vi "Measurement Logic.vi"() -> ()   [LabVIEW 2021, in "Line Transient_Channel Ganging.lvlib"]
uses:
  Line Transient_Channel Ganging.lvlib
  Measurement Results.ctl
  <instrlib>/niDCPower/nidcpower.llb/niDCPower Source Mode.ctl
  <instrlib>/niDCPower/nidcpower.llb/niDCPower Output Function.ctl
  <instrlib>/niDCPower/nidcpower.llb/niDCPower Wait For Event - Event.ctl
  shared subVIs/Triggers and Events/NIDCPower_channel_ganging - Configure Digital Edge Measure Trigger.vi
  shared subVIs/ctl/NIDCPower_channel_ganging - ctl - channel mode.ctl
  <instrlib>/niScope/Controls/niScope trigger slope.ctl
  <instrlib>/niScope/Acquire/Fetch/niScope Fetch WDT.vi
  <instrlib>/niScope/Configure/Trigger/niScope Configure Trigger Digital.vi
  <instrlib>/niScope/Utility/niScope Get Channel Name From String.vi
  shared subVIs/Triggers and Events/NIDCPower_channel_ganging - Configure Digital Edge Source Trigger.vi
  <vilib>/Plug-In SDKs/Measurements/Measure Call Context/Measure Call Context.lvclass
  Measurement Configuration.ctl
panel:
  in  "measurement configuration":T1={"Source master resource name"="", "Load master resource name"="", "Source slave resource names"=[], "Load slave resource names"=[], "Source system configuration"=enum."Parallel", "Source voltage level range"=20.0, "Source limit symmetry"=enum."Asymmetric", "Source current limit range"=25.0, "Source current limit low"=-0.6, "Source current limit high"=25.0, "Source transient response"=1038, "Source sense"=1009, "Source voltage level 1"=6.0, "Source sample rate"=1800000.0, "Source voltage level 2"=14.0, "Source voltage gain bandwidth"=2000.0, "Source voltage compensation frequency"=3530.0, "Source voltage pole-zero ratio"=2.0, "Load system configuration"=enum."Parallel", "Load current level"=1.0, "Load current level range"=80.0, "Load limit symmetry"=enum."Symmetric", "Load voltage limit range"=6.0, "Load voltage limit low"=0.0, "Load voltage limit high"=inf, "Load transient response"=1038, "Load sense"=1009, "DUT setup time"=1.0, "Load current gain bandwidth"=14000.0, "Load current compensation frequency"=180000.0, "Load current pole-zero ratio"=0.3, "Nominal output voltage"=1.0, "Source time delay 1"=6.0, "Source time delay 2"=0.005, "Source pulse duration"=0.005, "Source voltage falling slew rate"=24.0, "Source voltage rising slew rate"=24.0, "Scope resource name"="", "Scope output channel name"="0", "Scope sample rate"=1800000.0, "Scope probe attenuation"=1.0, "Scope vertical range"=10.0, "Scope vertical coupling"=enum."DC", "Scope enable/disable"=TRUE} {"Scope vertical range" format="%.2f"; "Scope probe attenuation" format="%.1f"; "Scope sample rate" step=1000000.0 format="%#.2g"; "Source voltage rising slew rate" format="%#_6p"; "Source time delay 1" format="%#_6p"; "Load sense" items=["Local"=1008, "Remote"=1009]; "Load transient response" items=["Slow"=1041, "Normal"=1038, "Fast"=1039, "Custom"=1042]; "Load voltage limit high" format="%#_6p"; "Load voltage limit low" format="%#_6p"; "Load voltage limit range" format="%#_6p"; "Load current level range" format="%#_6p"; "Source voltage level 1" format="%#_6p"; "Source sense" items=["Local"=1008, "Remote"=1009]; "Source transient response" items=["Slow"=1041, "Normal"=1038, "Fast"=1039, "Custom"=1042]; "Source current limit high" format="%#_6p"; "Source current limit low" format="%#_6p"; "Source current limit range" format="%#_6p"; "Source voltage level range" format="%#_6p"}
  out "measurement results":T2
  out "measure call context out":refnum<class "Measure Call Context.lvclass">
  in  "measure call context in":refnum<class "Measure Call Context.lvclass">
  out "error out":errorcluster
  in  "error in":errorcluster
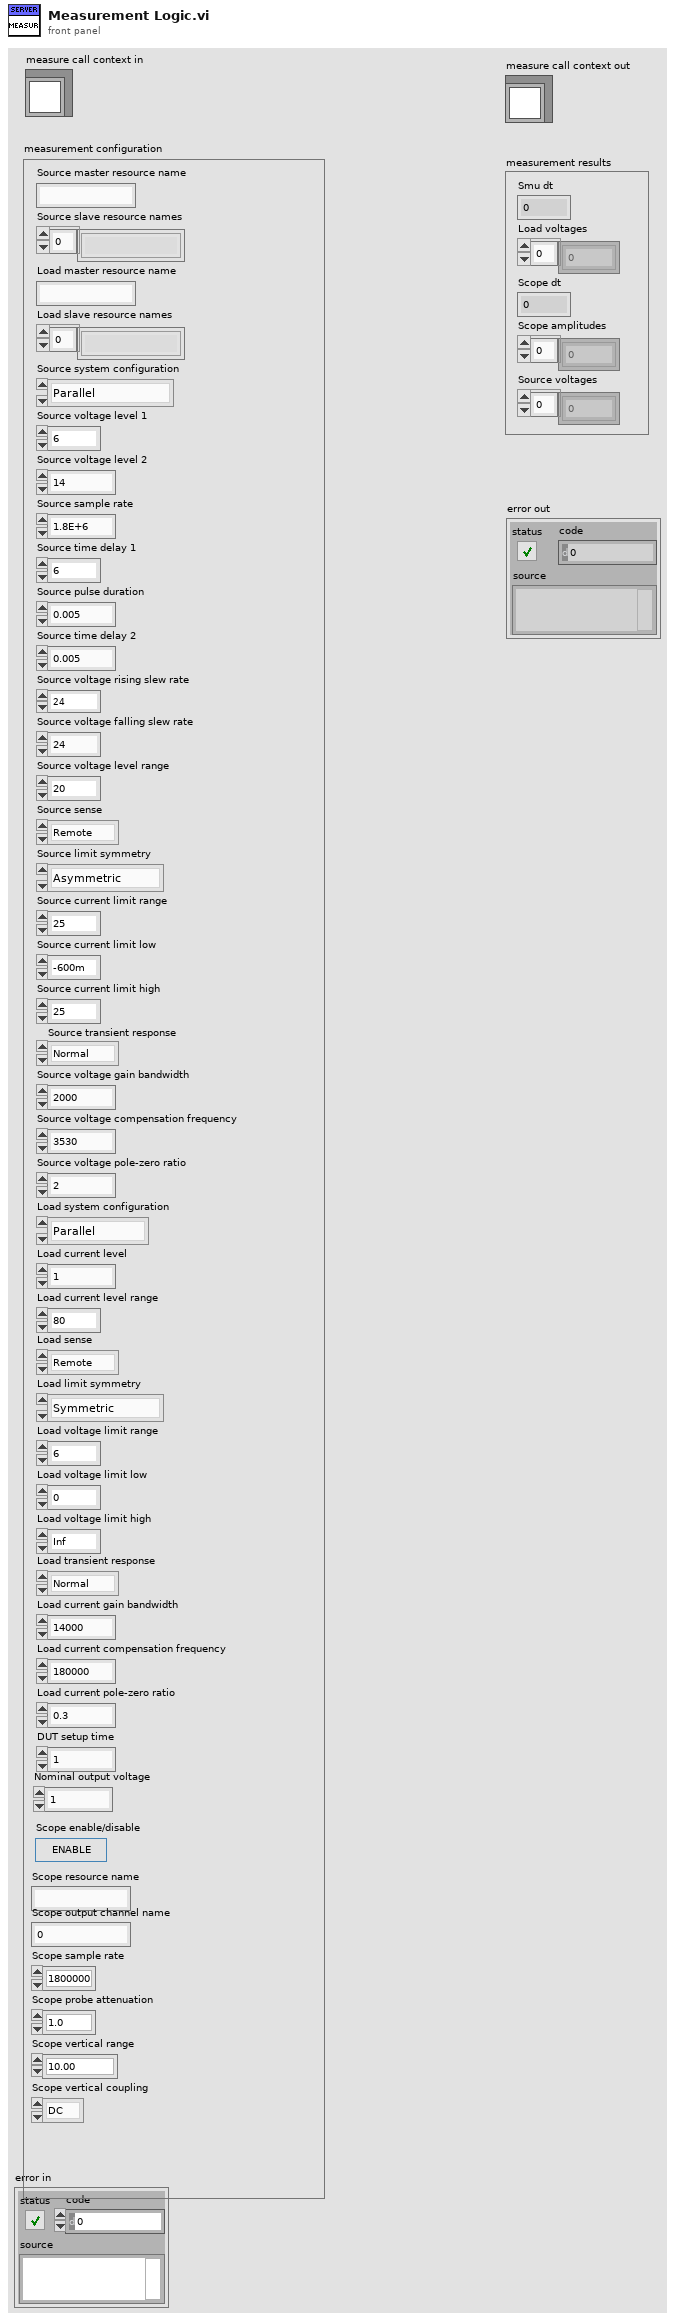
[diagram p1: front panel]
types:
  T1 = typedef "Line Transient_Channel Ganging.lvlib/Measurement Configuration.ctl" = cluster{"Source master resource name":string, "Load master resource name":string, "Source slave resource names":string[], "Load slave resource names":string[], "Source system configuration":enum32{"Series", "Parallel", "Manual"}, "Source voltage level range":dbl, "Source limit symmetry":enum32{"Symmetric", "Asymmetric"}, "Source current limit range":dbl, "Source current limit low":dbl, "Source current limit high":dbl, "Source transient response":i32, "Source sense":i32, "Source voltage level 1":dbl, "Source sample rate":dbl, "Source voltage level 2":dbl, "Source voltage gain bandwidth":dbl, "Source voltage compensation frequency":dbl, "Source voltage pole-zero ratio":dbl, "Load system configuration":enum32{"Series", "Parallel", "Manual"}, "Load current level":dbl, "Load current level range":dbl, "Load limit symmetry":enum32{"Symmetric", "Asymmetric"}, "Load voltage limit range":dbl, "Load voltage limit low":dbl, "Load voltage limit high":dbl, "Load transient response":i32, "Load sense":i32, "DUT setup time":dbl, "Load current gain bandwidth":dbl, "Load current compensation frequency":dbl, "Load current pole-zero ratio":dbl, "Nominal output voltage":dbl, "Source time delay 1":dbl, "Source time delay 2":dbl, "Source pulse duration":dbl, "Source voltage falling slew rate":dbl, "Source voltage rising slew rate":dbl, "Scope resource name":string, "Scope output channel name":string, "Scope sample rate":dbl, "Scope probe attenuation":dbl, "Scope vertical range":dbl, "Scope vertical coupling":enum32{"AC", "DC"}, "Scope enable/disable":bool}
  T2 = typedef "Line Transient_Channel Ganging.lvlib/Measurement Results.ctl" = cluster{"Smu dt":dbl, "Load voltages":dbl[], "Source voltages":dbl[], "Scope amplitudes":dbl[], "Scope dt":dbl}
  T3 = typedef "NIDCPower_channel_ganging - ctl - channel mode.ctl" = enum32{"Master", "Slave", "Slave - Inverted"}
  T4 = typedef "niDCPower Output Function.ctl" = i32
  T5 = typedef "niDCPower Source Mode.ctl" = i32
  T6 = typedef "niDCPower Wait For Event - Event.ctl" = i32
  T7 = typedef "NIDCPower_channel_ganging - ctl - channel def.ctl" = cluster{"resource name":refnum<k15>, "channels":string, "Channel Mode":T3}
  T8 = typedef "NIDCPower_channel_ganging - ctl - ganged session.ctl" = cluster{"Ganged Config":T9, "Session List":refnum<k15>[], "Session Mode":T3[], "Channel":string[]}
  T9 = typedef "NIDCPower_channel_ganging - ctl - ganged config.ctl" = enum32{"Series", "Parallel", "Manual"}
  T10 = typedef "niScope trigger slope.ctl" = i32
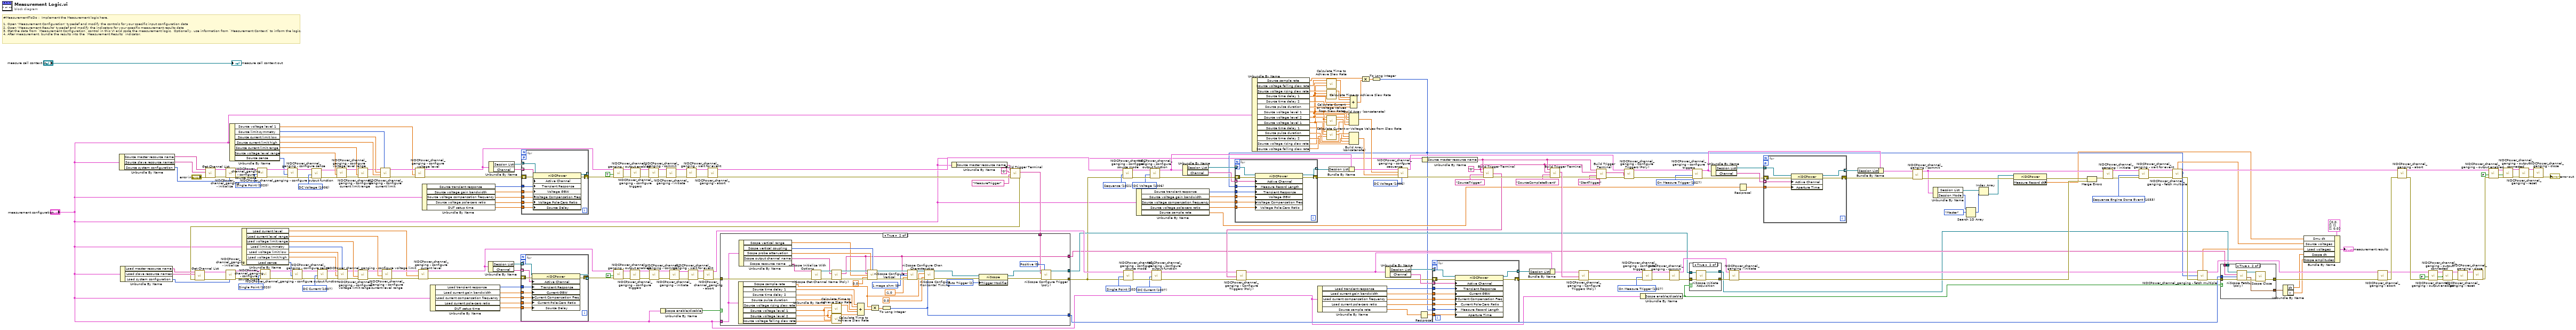
[diagram p0: block diagram]
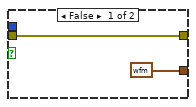
[diagram p2: hidden frame]
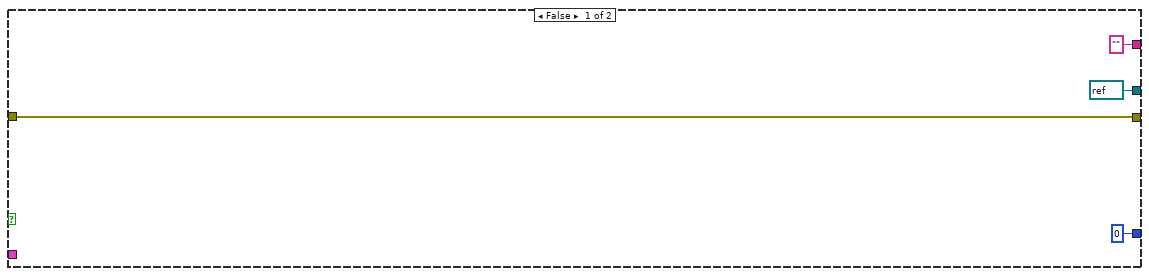
[diagram p4: hidden frame]
diagram:
  w100 = 1027 items=["Automatically after Source Complete"=1025, "On Demand"=1026, "On Measure Trigger"=1027] ("Measure When")
  w113 = T4 1006 items=["DC Voltage"=1006, "DC Current"=1007, "Pulse Voltage"=1049, "Pulse Current"=1050] ("output function")
  w96 = "0" ("Channel Name")
  w141 = 1027 items=["Automatically after Source Complete"=1025, "On Demand"=1026, "On Measure Trigger"=1027] ("Measure When")
  w138 = T4 1006 items=["DC Voltage"=1006, "DC Current"=1007, "Pulse Voltage"=1049, "Pulse Current"=1050] ("output function")
  w142 = T5 1021 items=["Single Point"=1020, "Sequence"=1021] ("source mode")
  w19 = T5 1020 items=["Single Point"=1020, "Sequence"=1021] ("source mode")
  w118 = T4 1007 items=["DC Voltage"=1006, "DC Current"=1007, "Pulse Voltage"=1049, "Pulse Current"=1050] ("output function")
  w147 = T6 1033 items=["Source Complete Event"=1030, "Measure Complete Event"=1031, "Sequence Iteration Complete Event"=1032, "Sequence Engine Done Event"=1033, "Pulse Complete Event"=1051, "Ready For Pulse Trigger Event"=1052] ("event")
  w151 = FALSE ("output enabled")
  w150 = FALSE ("output enabled")
  w223 = T4 1007 items=["DC Voltage"=1006, "DC Current"=1007, "Pulse Voltage"=1049, "Pulse Current"=1050] ("output function")
  w236 = T4 1006 items=["DC Voltage"=1006, "DC Current"=1007, "Pulse Voltage"=1049, "Pulse Current"=1050] ("output function")
  w255 = T5 1020 items=["Single Point"=1020, "Sequence"=1021] ("source mode")
  w256 = T5 1020 items=["Single Point"=1020, "Sequence"=1021] ("source mode")
  # "#MeasurementToDo :  Implement the Measurement logic here.\n\n1. Open 'Measurement Configuration' typedef and modify the controls for your specific input configuration data\n2. Open 'Measurement Results' typedef and modify the indicators for your specific measurement results data\n3. Get the data from `Measurement Configuration` control in this VI and code the measurement logic.  Optionally, use information from `Measurement Context` to inform the logic.\n4. After measurement, bundle the results into the `Measurement Results` indicator."
  n1 = Unbundle By Name("measurement configuration") -> ("Source master resource name"=w178:string, "Source slave resource names"=w177:string[], "Source system configuration"=w238:enum32{"Series", "Parallel", "Manual"})
  n2 = Unbundle By Name("measurement configuration") -> ("Load master resource name"=w174:string, "Load slave resource names"=w173:string[], "Load system configuration"=w237:enum32{"Series", "Parallel", "Manual"})
  n3 = call "Get Channel List.vi"("error in (no error)"="error in", "Slave resource names"=w177, "Master resouce name"=w178) -> ("error out"=w179:errorcluster, "Channel List"=w180:T7[])  [unwired: 7 in]
  n4 = call "NIDCPower_channel_ganging - initialize.vi"("Ganged Config"=w238, "error in (no error)"=w179, "Channel List"=w180) -> ("error out"=w257:errorcluster, "Ganged Session Out"=w258:T8)  [unwired: 7 in]
  n5 = Unbundle By Name("measurement configuration") -> ("Source voltage level 1"=w94:dbl, "Source limit symmetry"=w244:enum32{"Symmetric", "Asymmetric"}, "Source current limit low"=w245:dbl, "Source current limit high"=w246:dbl, "Source current limit range"=w247:dbl, "Source voltage level range"=w248:dbl, "Source sense"=w181:i32)
  n6 = Unbundle By Name("measurement configuration") -> ("Load current level"=w183:dbl, "Load current level range"=w239:dbl, "Load voltage limit range"=w240:dbl, "Load limit symmetry"=w243:enum32{"Symmetric", "Asymmetric"}, "Load voltage limit low"=w242:dbl, "Load voltage limit high"=w241:dbl, "Load sense"=w182:i32)
  n7 = call "NIDCPower_channel_ganging - configure source mode.vi"("error in (no error)"=w257, "source mode"=w256, "Ganged Session In"=w258) -> ("error out"=w221:errorcluster, "Ganged Session Out"=w222:T8)  [unwired: 7 in]
  n8 = call "NIDCPower_channel_ganging - configure sense.vi"("error in (no error)"=w221, "sense"=w181, "Ganged Session In"=w222) -> ("error out"=w219:errorcluster, "Ganged Session Out"=w220:T8)  [unwired: 7 in]
  n9 = call "NIDCPower_channel_ganging - configure output function.vi"("error in (no error)"=w219, "output function"=w236, "Ganged Session In"=w220) -> ("error out"=w217:errorcluster, "Ganged Session Out"=w218:T8)  [unwired: 7 in]
  n10 = call "NIDCPower_channel_ganging - configure voltage level range.vi"("error in (no error)"=w217, "voltage level range"=w248, "Ganged Session In"=w218) -> ("error out"=w232:errorcluster, "Ganged Session Out"=w235:T8)  [unwired: 7 in]
  n11 = call "NIDCPower_channel_ganging - configure current limit range.vi"("error in (no error)"=w232, "current limit range"=w247, "Ganged Session In"=w235) -> ("error out"=w231:errorcluster, "Ganged Session Out"=w234:T8)  [unwired: 7 in]
  n12 = call "NIDCPower_channel_ganging - configure current limit.vi"("Limit Symmetry"=w244, "error in (no error)"=w231, "Current limit/hi"=w246, "Current limit lo"=w245, "Ganged Session In"=w234) -> ("error out"=w230:errorcluster, "Ganged Session Out"=w233:T8)  [unwired: 5 in]
  n13 = call "NIDCPower_channel_ganging - configure voltage level.vi"("error in (no error)"=w230, "voltage level"=w94, "Ganged Session In"=w233) -> ("error out"=w192:errorcluster, "Ganged Session Out"=w186:T8)  [unwired: 7 in]
  n14 = Unbundle By Name("measurement configuration") -> ("Source transient response"=w172:i32, "Source voltage gain bandwidth"=w168:dbl, "Source voltage compensation frequency"=w167:dbl, "Source voltage pole-zero ratio"=w166:dbl, "DUT setup time"=w169:dbl)
  n15 = Unbundle By Name("measurement configuration") -> ("Load transient response"=w171:i32, "Load current gain bandwidth"=w165:dbl, "Load current compensation frequency"=w164:dbl, "Load current pole-zero ratio"=w163:dbl, "DUT setup time"=w170:dbl)
  n16 = Unbundle By Name(w186) -> ("Session List"=w190:refnum<k15>[], "Channel"=w189:string[])
  n17 = for {
    tunnel: [w269] -> _ mode=indexing
    shift-right: [w267] -> w191
    shift-left: w192 -> [w268]
    workers-P: _ -> [_]
    tunnel: w190 -> [w266] mode=indexing
    tunnel: w189 -> [w265] mode=indexing
    tunnel: w172 -> [w264]
    tunnel: w169 -> [w263]
    tunnel: w168 -> [w262]
    tunnel: w167 -> [w261]
    tunnel: w166 -> [w260]
    n18 = property class="niDCPower"(reference=w266, error in=w268, "Active Channel"=w265, "Transient Response"=w264, "Voltage GBW"=w262, "Voltage Compensation Freq"=w261, "Voltage Pole-Zero Ratio"=w260, "Source Delay"=w263) -> (reference out=w269:refnum<k15>, error out=w267:errorcluster)
  }
  n19 = call "NIDCPower_channel_ganging - output enabled.vi"("error in (no error)"=w191, "output enabled"=TRUE, "Ganged Session In"=w186) -> ("error out"=w195:errorcluster, "Ganged Session Out"=w196:T8)  [unwired: 7 in]
  n20 = call "NIDCPower_channel_ganging - configure triggers.vi"("error in (no error)"=w195, "Ganged Session In"=w196) -> ("error out"=w193:errorcluster, "Ganged Session Out"=w194:T8)  [unwired: 8 in]
  n21 = call "NIDCPower_channel_ganging - commit.vi"("error in (no error)"=w193, "Ganged Session In"=w194) -> ("error out"=w202:errorcluster, "Ganged Session Out"=w201:T8)  [unwired: 8 in]
  n22 = Unbundle By Name("measurement configuration") -> ("Scope enable/disable"=w13:bool)
  n23 = call "NIDCPower_channel_ganging - initiate.vi"("error in (no error)"=w202, "Ganged Session In"=w201) -> ("error out"=w204:errorcluster, "Ganged Session Out"=w203:T8)  [unwired: 8 in]
  n24 = call "NIDCPower_channel_ganging - wait for event.vi"("error in (no error)"=w204, "Ganged Session in"=w203) -> ("error out"=w206:errorcluster, "Ganged Session Out"=w205:T8)  [unwired: 8 in]
  n25 = call "NIDCPower_channel_ganging - abort.vi"("error in (no error)"=w206, "Ganged Session In"=w205) -> ("error out"=w33:errorcluster, "Ganged Session Out"=w31:T8)  [unwired: 8 in]
  n26 = Unbundle By Name("measurement configuration") -> ("Source master resource name"=w30:string)
  n27 = call "Build Trigger Terminal.vi"("error in (no error)"=w33, "Trigger/Event Name"="MeasureTrigger", "Channel Name"="0", "Resource Name"=w30) -> ("error out"=w34:errorcluster, "Terminal Name"=w18:string)  [unwired: 6 in]
  n28 = call "Get Channel List.vi"("error in (no error)"=w34, "Slave resource names"=w173, "Master resouce name"=w174) -> ("error out"=w176:errorcluster, "Channel List"=w175:T7[])  [unwired: 7 in]
  n29 = call "NIDCPower_channel_ganging - initialize.vi"("Ganged Config"=w237, "error in (no error)"=w176, "Channel List"=w175) -> ("error out"=w254:errorcluster, "Ganged Session Out"=w253:T8)  [unwired: 7 in]
  n30 = call "NIDCPower_channel_ganging - configure source mode.vi"("error in (no error)"=w254, "source mode"=w255, "Ganged Session In"=w253) -> ("error out"=w215:errorcluster, "Ganged Session Out"=w216:T8)  [unwired: 7 in]
  n31 = call "NIDCPower_channel_ganging - configure sense.vi"("error in (no error)"=w215, "sense"=w182, "Ganged Session In"=w216) -> ("error out"=w213:errorcluster, "Ganged Session Out"=w214:T8)  [unwired: 7 in]
  n32 = call "NIDCPower_channel_ganging - configure output function.vi"("error in (no error)"=w213, "output function"=w223, "Ganged Session In"=w214) -> ("error out"=w251:errorcluster, "Ganged Session Out"=w252:T8)  [unwired: 7 in]
  n33 = call "NIDCPower_channel_ganging - configure voltage limit.vi"("Limit Symmetry"=w243, "error in (no error)"=w251, "voltage limit/hi"=w241, "voltage limit lo"=w242, "Ganged Session In"=w252) -> ("error out"=w228:errorcluster, "Ganged Session Out"=w229:T8)  [unwired: 5 in]
  n34 = call "NIDCPower_channel_ganging - configure voltage limit range.vi"("error in (no error)"=w228, "voltage level range"=w240, "Ganged Session In"=w229) -> ("error out"=w226:errorcluster, "Ganged Session Out"=w227:T8)  [unwired: 7 in]
  n35 = call "NIDCPower_channel_ganging - configure current level range.vi"("error in (no error)"=w226, "current level range"=w239, "Ganged Session In"=w227) -> ("error out"=w224:errorcluster, "Ganged Session Out"=w225:T8)  [unwired: 7 in]
  n36 = call "NIDCPower_channel_ganging - configure current level.vi"("error in (no error)"=w224, "current level"=w183, "Ganged Session In"=w225) -> ("error out"=w188:errorcluster, "Ganged Session Out"=w60:T8)  [unwired: 7 in]
  n37 = Unbundle By Name(w60) -> ("Session List"=w185:refnum<k15>[], "Channel"=w184:string[])
  n38 = for {
    tunnel: [w279] -> _ mode=indexing
    shift-right: [w277] -> w187
    shift-left: w188 -> [w278]
    workers-P: _ -> [_]
    tunnel: w185 -> [w276] mode=indexing
    tunnel: w184 -> [w275] mode=indexing
    tunnel: w171 -> [w274]
    tunnel: w170 -> [w273]
    tunnel: w165 -> [w272]
    tunnel: w164 -> [w271]
    tunnel: w163 -> [w270]
    n39 = property class="niDCPower"(reference=w276, error in=w278, "Active Channel"=w275, "Transient Response"=w274, "Current GBW"=w272, "Current Compensation Freq"=w271, "Current Pole-Zero Ratio"=w270, "Source Delay"=w273) -> (reference out=w279:refnum<k15>, error out=w277:errorcluster)
  }
  n40 = call "NIDCPower_channel_ganging - output enabled.vi"("error in (no error)"=w187, "output enabled"=TRUE, "Ganged Session In"=w60) -> ("error out"=w199:errorcluster, "Ganged Session Out"=w200:T8)  [unwired: 7 in]
  n41 = call "NIDCPower_channel_ganging - configure triggers.vi"("error in (no error)"=w199, "Ganged Session In"=w200) -> ("error out"=w197:errorcluster, "Ganged Session Out"=w198:T8)  [unwired: 8 in]
  n42 = call "NIDCPower_channel_ganging - commit.vi"("error in (no error)"=w197, "Ganged Session In"=w198) -> ("error out"=w211:errorcluster, "Ganged Session Out"=w212:T8)  [unwired: 8 in]
  n43 = call "NIDCPower_channel_ganging - initiate.vi"("error in (no error)"=w211, "Ganged Session In"=w212) -> ("error out"=w209:errorcluster, "Ganged Session Out"=w210:T8)  [unwired: 8 in]
  n44 = call "NIDCPower_channel_ganging - wait for event.vi"("error in (no error)"=w209, "Ganged Session in"=w210) -> ("error out"=w207:errorcluster, "Ganged Session Out"=w208:T8)  [unwired: 8 in]
  n45 = call "NIDCPower_channel_ganging - abort.vi"("error in (no error)"=w207, "Ganged Session In"=w208) -> ("error out"=w20:errorcluster, "Ganged Session Out"=w105:T8)  [unwired: 8 in]
  n46 = case shown="True" w13 {
    tunnel: w20 -> [w283 w293]
    tunnel: "measurement configuration" -> [_ w292]
    tunnel: [w283 w291] -> w2
    tunnel: w18 -> [_ w290]
    tunnel: ["" ("channel name") w288] -> w16
    tunnel: [refnum<k15> refnum ("instrument handle out") w287] -> w17
    tunnel: [0 w286] -> w14
    frame False {
    }
    frame True {
      w314 = 2 items=["None"=1, "Auto Trigger"=2] ("Trigger Modifier")
      w307 = u32 0 items=["1 mega ohm"=0, "50 ohms"=2] ("Input Impedance")
      w311 = T10 0 items=["Positive", "Negative"] ("trigger slope")
      n47 = Unbundle By Name(w292) -> ("Scope sample rate"=w284:dbl, "Source time delay 1"=w305:dbl, "Source time delay 2"=w304:dbl, "Source pulse duration"=w303:dbl, "Source voltage rising slew rate"=w301:dbl, "Source voltage level 1"=w296:dbl, "Source voltage level 2"=w297:dbl, "Source voltage falling slew rate"=w299:dbl)
      n48 = Unbundle By Name(w292) -> ("Scope vertical range"=w285:dbl, "Scope vertical coupling"=w309:enum32{"AC", "DC"}, "Scope probe attenuation"=w310:dbl, "Scope output channel name"=w308:string, "Scope resource name"=w289:string)
      n49 = call <instrlib>:"niScope Initialize With Options.vi"("resource name"=w289, "error in"=w293) -> ("instrument handle"=w325:refnum<k15>, "error out"=w324:errorcluster)  [unwired: 12 in]
      n50 = call-poly <instrlib>:"niScope Get Channel Name (Poly).vi"("instrument handle"=w325, "index"=w308, "error in"=w324) -> ("instrument handle out"=w313:refnum<k15>, "channel name"=w288:string, "error out"=w312:errorcluster)  [unwired: 10 in]
      n51 = call "Calculate Time to Achieve Slew Rate.vi"("Current/voltage set point 2"=w297, "Current/voltage set point 1"=w296, "Current/voltage slew rate"=w301) -> ("Calculated time"=w300:dbl)  [unwired: 8 in]
      n52 = call "Calculate Time to Achieve Slew Rate.vi"("Current/voltage set point 2"=w296, "Current/voltage set point 1"=w297, "Current/voltage slew rate"=w299) -> ("Calculated time"=w298:dbl)  [unwired: 8 in]
      n53 = Compound Arithmetic op=ADD(w305, w304, w303, w300, w298) -> (w294:dbl)
      n54 = call <instrlib>:"niScope Configure Vertical.vi"("instrument handle"=w313, "probe attenuation"=w310, "vertical coupling"=w309, "channels"=w288, "vertical range"=w285, "vertical offset"=0.0, "error in"=w312) -> ("instrument handle out"=w323:refnum<k15>, "error out"=w322:errorcluster)  [unwired: 7 in]
      n55 = Compound Arithmetic op=MULTIPLY(w284, w294) -> (w295:dbl)
      n56 = To Long Integer(number=w295) -> (32bit integer=w286:i32)
      n57 = call <instrlib>:"niScope Configure Chan Characteristics.vi"("instrument handle"=w323, "channels"=w288, "input impedance"=w307, "maximum input frequency"=-1.0 ("Maximum Input Frequency"), "error in"=w322) -> ("instrument handle out"=w320:refnum<k15>, "error out"=w321:errorcluster)  [unwired: 9 in]
      n58 = call <instrlib>:"niScope Configure Horizontal Timing.vi"("instrument handle"=w320, "min sample rate"=w284, "reference position"=0.0 ("Reference Position"), "error in"=w321, "min record length"=w286) -> ("instrument handle out"=w317:refnum<k15>, "error out"=w316:errorcluster)  [unwired: 9 in]
      n59 = property on="Property Node" class="niScope"(reference=w317, error in=w316, "Trigger Modifier"=w314) -> (reference out=w302:refnum<k15>, error out=w315:errorcluster)
      n60 = call-poly <instrlib>:"niScope Configure Trigger (poly).vi"("instrument handle"=w302, "trigger slope"=w311, "trigger source"=w290, "error in"=w315) -> ("instrument handle out"=w287:refnum<k15>, "error out"=w291:errorcluster)  [unwired: 10 in]
    }
  }
  n61 = call "NIDCPower_channel_ganging - configure source mode.vi"("error in (no error)"=w2, "source mode"=w142, "Ganged Session In"=w31) -> ("error out"=w143:errorcluster, "Ganged Session Out"=w144:T8)  [unwired: 7 in]
  n62 = call "NIDCPower_channel_ganging - configure source mode.vi"("error in (no error)"=w2, "source mode"=w19, "Ganged Session In"=w105) -> ("error out"=w146:errorcluster, "Ganged Session Out"=w145:T8)  [unwired: 7 in]
  n63 = Unbundle By Name("measurement configuration") -> ("Source transient response"=w114:i32, "Source voltage gain bandwidth"=w111:dbl, "Source voltage compensation frequency"=w110:dbl, "Source voltage pole-zero ratio"=w109:dbl, "Source sample rate"=w24:dbl)
  n64 = call "NIDCPower_channel_ganging - configure output function.vi"("error in (no error)"=w143, "output function"=w138, "Ganged Session In"=w144) -> ("error out"=w139:errorcluster, "Ganged Session Out"=w140:T8)  [unwired: 7 in]
  n65 = call "NIDCPower_channel_ganging - configure output function.vi"("error in (no error)"=w146, "output function"=w118, "Ganged Session In"=w145) -> ("error out"=w55:errorcluster, "Ganged Session Out"=w53:T8)  [unwired: 7 in]
  n66 = Unbundle By Name(w140) -> ("Session List"=w162:refnum<k15>[], "Channel"=w128:string[])
  n67 = Unbundle By Name("measurement configuration") -> ("Source sample rate"=w86:dbl, "Source voltage falling slew rate"=w84:dbl, "Source voltage rising slew rate"=w82:dbl, "Source time delay 1"=w92:dbl, "Source time delay 2"=w85:dbl, "Source pulse duration"=w90:dbl, "Source voltage level 1"=w80:dbl, "Source voltage level 2"=w76:dbl, "Source voltage level 1"=w75:dbl, "Source time delay 1"=w89:dbl, "Source pulse duration"=w88:dbl, "Source time delay 2"=w87:dbl, "Source voltage rising slew rate"=w79:dbl, "Source voltage falling slew rate"=w74:dbl)
  n68 = Unbundle By Name("measurement configuration") -> ("Load transient response"=w112:i32, "Load current gain bandwidth"=w108:dbl, "Load current compensation frequency"=w107:dbl, "Load current pole-zero ratio"=w106:dbl, "Source sample rate"=w59:dbl)
  n69 = call "Calculate Time to Achieve Slew Rate.vi"("Current/voltage set point 2"=w80, "Current/voltage set point 1"=w76, "Current/voltage slew rate"=w84) -> ("Calculated time"=w83:dbl)  [unwired: 8 in]
  n70 = call "Calculate Time to Achieve Slew Rate.vi"("Current/voltage set point 2"=w76, "Current/voltage set point 1"=w80, "Current/voltage slew rate"=w82) -> ("Calculated time"=w81:dbl)  [unwired: 8 in]
  n71 = call "Calculate Current or Voltage Values from Slew Rate.vi"("Current/voltage slew rate"=w79, "Current/voltage end point"=w76, "Current/voltage start point"=w80) -> ("Source delays"=w77:dbl[], "Current/voltage values"=w78:dbl[])  [unwired: 7 in]
  n72 = call "Calculate Current or Voltage Values from Slew Rate.vi"("Current/voltage slew rate"=w74, "Current/voltage end point"=w75, "Current/voltage start point"=w76) -> ("Source delays"=w72:dbl[], "Current/voltage values"=w73:dbl[])  [unwired: 7 in]
  n73 = Build Array (concatenate)(w80, w78, w76, w73, w75) -> (w71:dbl[])
  n74 = Build Array (concatenate)(w89, w77, w88, w72, w87) -> (w70:dbl[])
  n75 = Compound Arithmetic op=ADD(w83, w81, w92, w85, w90) -> (w91:dbl)
  n76 = Compound Arithmetic op=MULTIPLY(w86, w91) -> (w93:dbl)
  n77 = To Long Integer(number=w93) -> (32bit integer=w3:i32)
  n78 = for {
    tunnel: [w335] -> w161 mode=indexing
    shift-right: [w333] -> w116
    shift-left: w139 -> [w334]
    workers-P: _ -> [_]
    tunnel: w162 -> [w332] mode=indexing
    tunnel: w128 -> [w327] mode=indexing
    tunnel: w114 -> [w331]
    tunnel: w111 -> [w330]
    tunnel: w110 -> [w329]
    tunnel: w109 -> [w328]
    tunnel: w3 -> [w326]
    n79 = property class="niDCPower"(reference=w332, error in=w334, "Active Channel"=w327, "Measure Record Length"=w326, "Transient Response"=w331, "Voltage GBW"=w330, "Voltage Compensation Freq"=w329, "Voltage Pole-Zero Ratio"=w328) -> (reference out=w335:refnum<k15>, error out=w333:errorcluster)
  }
  n80 = Bundle By Name(cluster=w140, "Session List"=w161) -> (w117:T8)
  n81 = call "NIDCPower_channel_ganging - confgure sequence.vi"("output function"=w113, "error in (no error)"=w116, "Source Delays"=w70, "Values"=w71, "Ganged Session In"=w117) -> ("error out"=w115:errorcluster, "Ganged Session Out"=w102:T8)  [unwired: 5 in]
  n82 = Reciprocal(x=w59) -> (1/x=w58:dbl)
  n83 = Unbundle By Name("measurement configuration") -> ("Source master resource name"=w97:string)
  n84 = call "Build Trigger Terminal.vi"("error in (no error)"=w115, "Trigger/Event Name"="SourceTrigger", "Channel Name"=w96, "Resource Name"=w97) -> ("error out"=w124:errorcluster, "Terminal Name"=w51:string)  [unwired: 6 in]
  n85 = call-poly "NIDCPower_channel_ganging - Configure Triggers (Poly).vi"("error in (no error)"=w55, "output terminal"=w51, "Ganged Session in"=w53) -> ("error out"=w54:errorcluster, "Ganged Session out"=w52:T8)  [unwired: 7 in]
  n86 = Unbundle By Name(w52) -> ("Session List"=w127:refnum<k15>[], "Channel"=w126:string[])
  n87 = for {
    tunnel: [w346] -> w125 mode=indexing
    shift-right: [w344] -> w57
    shift-left: w54 -> [w345]
    workers-P: _ -> [_]
    tunnel: w127 -> [w343] mode=indexing
    tunnel: w126 -> [w342] mode=indexing
    tunnel: w112 -> [w341]
    tunnel: w108 -> [w340]
    tunnel: w107 -> [w339]
    tunnel: w106 -> [w338]
    tunnel: w3 -> [w337]
    tunnel: w58 -> [w336]
    n88 = property class="niDCPower"(reference=w343, error in=w345, "Active Channel"=w342, "Transient Response"=w341, "Current GBW"=w340, "Current Compensation Freq"=w339, "Current Pole-Zero Ratio"=w338, "Measure Record Length"=w337, "Aperture Time"=w336) -> (reference out=w346:refnum<k15>, error out=w344:errorcluster)
  }
  n89 = Bundle By Name(cluster=w52, "Session List"=w125) -> (w56:T8)
  n90 = call "Build Trigger Terminal.vi"("error in (no error)"=w124, "Trigger/Event Name"="SourceCompleteEvent", "Channel Name"=w96, "Resource Name"=w97) -> ("error out"=w99:errorcluster, "Terminal Name"=w119:string)  [unwired: 6 in]
  n91 = call-poly "NIDCPower_channel_ganging - Configure Triggers (Poly).vi"("error in (no error)"=w57, "output terminal"=w119, "Ganged Session in"=w56) -> ("error out"=w120:errorcluster, "Ganged Session out"=w121:T8)  [unwired: 7 in]
  n92 = call "Build Trigger Terminal.vi"("error in (no error)"=w99, "Trigger/Event Name"="StartTrigger" ("Source master resource name"), "Channel Name"=w96, "Resource Name"=w97) -> ("error out"=w104:errorcluster, "Terminal Name"=w95:string)  [unwired: 6 in]
  n93 = call-poly "NIDCPower_channel_ganging - Configure Triggers (Poly).vi"("error in (no error)"=w104, "output terminal"=w95, "Ganged Session in"=w102) -> ("error out"=w103:errorcluster, "Ganged Session out"=w101:T8)  [unwired: 7 in]
  n94 = Unbundle By Name("measurement configuration") -> ("Scope enable/disable"=w12:bool)
  n95 = call "NIDCPower_channel_ganging - configure triggers.vi"("error in (no error)"=w120, "Measure When"=w141, "Ganged Session In"=w121) -> ("error out"=w37:errorcluster, "Ganged Session Out"=w36:T8)  [unwired: 7 in]
  n96 = call "NIDCPower_channel_ganging - commit.vi"("error in (no error)"=w37, "Ganged Session In"=w36) -> ("error out"=w28:errorcluster, "Ganged Session Out"=w35:T8)  [unwired: 8 in]
  n97 = case shown="True" w12 {
    tunnel: w28 -> [w347 w350]
    tunnel: [w347 w351] -> w27
    tunnel: w17 -> [_ w349]
    tunnel: [_ w348] -> w15
    frame False {
    }
    frame True {
      n98 = call <instrlib>:"niScope Initiate Acquisition.vi"("instrument handle"=w349, "error in"=w350) -> ("instrument handle out"=w348:refnum<k15>, "error out"=w351:errorcluster)  [unwired: 12 in]
    }
  }
  n99 = call "NIDCPower_channel_ganging - configure triggers.vi"("error in (no error)"=w103, "Measure When"=w100, "Ganged Session In"=w101) -> ("error out"=w65:errorcluster, "Ganged Session Out"=w66:T8)  [unwired: 7 in]
  n100 = Unbundle By Name(w66) -> ("Session List"=w69:refnum<k15>[], "Channel"=w67:string[])
  n101 = call "NIDCPower_channel_ganging - initiate.vi"("error in (no error)"=w27, "Ganged Session In"=w35) -> ("error out"=w148:errorcluster, "Ganged Session Out"=w50:T8)  [unwired: 8 in]
  n102 = Reciprocal(x=w24) -> (1/x=w23:dbl)
  n103 = for {
    tunnel: [w352] -> w68 mode=indexing
    shift-right: [w356] -> w41
    shift-left: w65 -> [w357]
    workers-P: _ -> [_]
    tunnel: w69 -> [w355] mode=indexing
    tunnel: w67 -> [w354] mode=indexing
    tunnel: w23 -> [w353]
    n104 = property class="niDCPower"(reference=w355, error in=w357, "Active Channel"=w354, "Aperture Time"=w353) -> (reference out=w352:refnum<k15>, error out=w356:errorcluster)
  }
  n105 = Bundle By Name(cluster=w66, "Session List"=w68) -> (w40:T8)
  n106 = call "NIDCPower_channel_ganging - commit.vi"("error in (no error)"=w41, "Ganged Session In"=w40) -> ("error out"=w47:errorcluster, "Ganged Session Out"=w39:T8)  [unwired: 8 in]
  n107 = Unbundle By Name(w39) -> ("Session List"=w45:refnum<k15>[], "Session Mode"=w44:T3[])
  n108 = Search 1D Array(1D array=w44, element=NIDCPower_channel_ganging_-_ctl_-_channel_mode."Master") -> (index of element=w42:i32)  [unwired: 1 in]
  n109 = Index Array(array=w45, index=w42) -> (element=w46:refnum<k15>)
  n110 = property class="niDCPower"(reference=w46, error in=w47) -> (error out=w38:errorcluster, "Measure Record dt"=w9:dbl)  [unwired: 1 out]
  n111 = Merge Errors(w38, w148) -> (w149:errorcluster)
  n112 = call "NIDCPower_channel_ganging - initiate.vi"("error in (no error)"=w149, "Ganged Session In"=w39) -> ("error out"=w137:errorcluster, "Ganged Session Out"=w49:T8)  [unwired: 8 in]
  n113 = call "NIDCPower_channel_ganging - wait for event.vi"("error in (no error)"=w137, "event"=w147, "Ganged Session in"=w49) -> ("error out"=w63:errorcluster, "Ganged Session Out"=w48:T8)  [unwired: 7 in]
  n114 = call "NIDCPower_channel_ganging - fetch multiple.vi"("Ganged Session In"=w48, "Count"=w3, "error in (no error)"=w63) -> ("Ganged Voltage Measurement"=w4:dbl[], "Ganged Session Out"=w64:T8, "error out"=w62:errorcluster)  [unwired: 5 in, 5 out]
  n115 = call "NIDCPower_channel_ganging - fetch multiple.vi"("Ganged Session In"=w50, "Count"=w3, "error in (no error)"=w62) -> ("Ganged Voltage Measurement"=w8:dbl[], "Ganged Session Out"=w61:T8, "error out"=w26:errorcluster)  [unwired: 5 in, 5 out]
  n116 = case shown="True" w12 {
    tunnel: w26 -> [w359 w367]
    tunnel: [w359 w366] -> w25
    tunnel: w16 -> [_ w363]
    tunnel: w15 -> [_ w362]
    tunnel: w14 -> [_ w361]
    tunnel: [waveform(dbl) {"t0"=timestamp(0 s since 1904-01-01), "dt"=1.0, "Y"=[]} ("wfm") w360] -> w7
    frame False {
    }
    frame True {
      n117 = call-poly <instrlib>:"niScope Fetch (poly).vi"("error in"=w367, "numSamples"=w361, "channels"=w363, "instrument handle"=w362) -> ("error out"=w365:errorcluster, "wfm"=w360:waveform(dbl), "instrument handle out"=w364:refnum<k15>)  [unwired: 4 in, 1 out]
      n118 = call <instrlib>:"niScope Close.vi"("instrument handle"=w364, "error in"=w365) -> ("error out"=w366:errorcluster)  [unwired: 13 in]
    }
  }
  n119 = Unbundle By Name(w7) -> ("dt"=w6:dbl, "Y"=w5:dbl[])
  n120 = Bundle By Name(cluster=T2 {"Smu dt"=0.0, "Load voltages"=[], "Source voltages"=[], "Scope amplitudes"=[], "Scope dt"=0.0} ("Measurement Results"), "Smu dt"=w9, "Source voltages"=w4, "Load voltages"=w8, "Scope dt"=w6, "Scope amplitudes"=w5) -> (→"measurement results":T2)
  n121 = call "NIDCPower_channel_ganging - abort.vi"("error in (no error)"=w25, "Ganged Session In"=w61) -> ("error out"=w160:errorcluster, "Ganged Session Out"=w156:T8)  [unwired: 8 in]
  n122 = call "NIDCPower_channel_ganging - abort.vi"("error in (no error)"=w160, "Ganged Session In"=w64) -> ("error out"=w159:errorcluster, "Ganged Session Out"=w152:T8)  [unwired: 8 in]
  n123 = call "NIDCPower_channel_ganging - output enabled.vi"("error in (no error)"=w159, "output enabled"=w151, "Ganged Session In"=w156) -> ("error out"=w157:errorcluster, "Ganged Session Out"=w158:T8)  [unwired: 7 in]
  n124 = call "NIDCPower_channel_ganging - output connected.vi"("error in (no error)"=w157, "output enabled"=w151, "Ganged Session In"=w158) -> ("error out"=w136:errorcluster, "Ganged Session Out"=w135:T8)  [unwired: 7 in]
  n125 = call "NIDCPower_channel_ganging - reset.vi"("error in (no error)"=w136, "Ganged Session In"=w135) -> ("error out"=w133:errorcluster, "Ganged Session Out"=w134:T8)  [unwired: 8 in]
  n126 = call "NIDCPower_channel_ganging - close.vi"("error in (no error)"=w133, "Ganged Session In"=w134) -> ("error out"=w153:errorcluster)  [unwired: 9 in]
  n127 = call "NIDCPower_channel_ganging - output enabled.vi"("error in (no error)"=w153, "output enabled"=w150, "Ganged Session In"=w152) -> ("error out"=w155:errorcluster, "Ganged Session Out"=w154:T8)  [unwired: 7 in]
  n128 = call "NIDCPower_channel_ganging - output connected.vi"("error in (no error)"=w155, "output enabled"=w150, "Ganged Session In"=w154) -> ("error out"=w131:errorcluster, "Ganged Session Out"=w132:T8)  [unwired: 7 in]
  n129 = call "NIDCPower_channel_ganging - reset.vi"("error in (no error)"=w131, "Ganged Session In"=w132) -> ("error out"=w129:errorcluster, "Ganged Session Out"=w130:T8)  [unwired: 8 in]
  n130 = call "NIDCPower_channel_ganging - close.vi"("error in (no error)"=w129, "Ganged Session In"=w130) -> ("error out"=→"error out":errorcluster)  [unwired: 9 in]
  "measure call context out" <- "measure call context in"
